vi "From WAMP Message.vi"(8 "error in (no error)":errorcluster, 11 "JSONMessage":refnum<class "JSONMessage.lvclass">) -> (0 "error out":errorcluster, 3 "HandlePublished JSON out":refnum<class "HandlePublished JSON.lvclass">)   [LabVIEW 2020, in "wamplv.lvlib" / "HandlePublished JSON.lvclass"]
uses:
  HandlePublished JSON.lvclass
  SerialisedMessages/JSONMessage/JSONMessage.lvclass
  HandlePublished JSON.lvclass/HandlePublished JSON.ctl
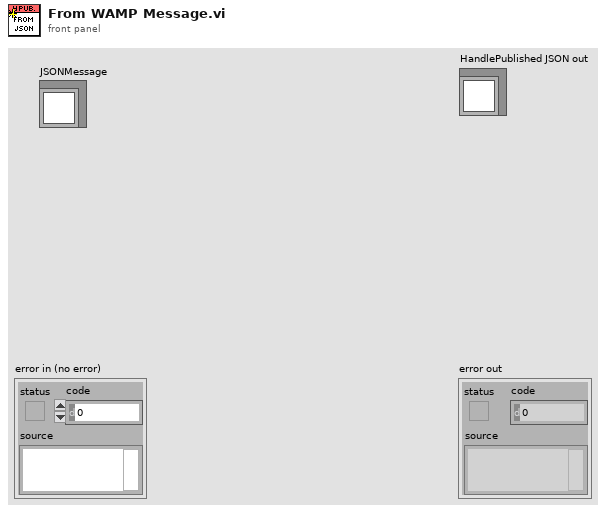
[diagram p1: front panel]
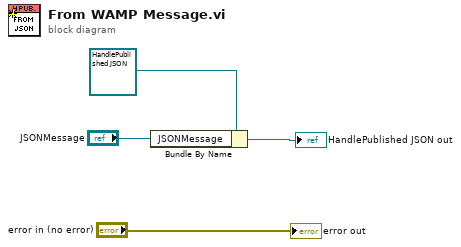
[diagram p0: block diagram]
diagram:
  n1 = Bundle By Name(cluster=refnum<class "HandlePublished JSON.lvclass"> refnum ("wamplv.lvlib:HandlePublished JSON.lvclass"), "JSONMessage"="JSONMessage") -> (→"HandlePublished JSON out":refnum<class "HandlePublished JSON.lvclass">)
  "error out" <- "error in (no error)"
